vi "waitForRisEdgeTest.vi"(6 "stop":bool, 9 "delay(ticks)":u32) -> (3 "i":i32)   [LabVIEW 2014]
uses:
  <vilib>/eio/EIONode/EIONode.xnode
  <vilib>/rvi/eio/common/nirviEmuTemplateMethod_errors.vi
panel:
  in  "trigSelect":u16 format="%016b"
  in  "waitbeforeNextGo(Ticks)":u32 caption="waitBeforeNextGo(Ticks)"
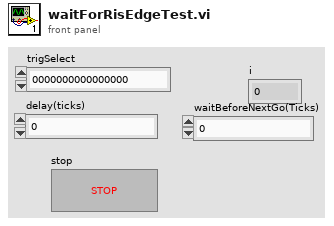
[diagram p1: front panel]
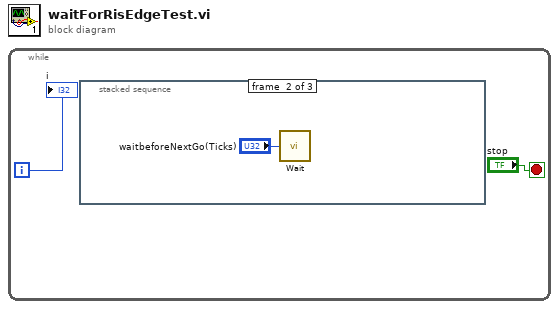
[diagram p0: block diagram]
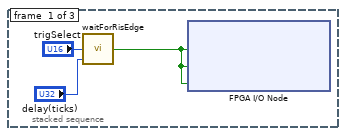
[diagram p2: hidden frame]
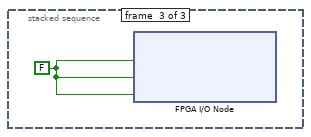
[diagram p3: hidden frame]
diagram:
  n1 = while {
    i -> [w1]
    stop <- "stop" stop-if-true
    n2 = stacked-sequence {
      frame #0 {
        n3 = call "waitForRisEdge.vi"("delay(ticks)"="delay(ticks)", "MCSSelectTrigger"="trigSelect") -> ("out"=w3:bool)  [unwired: 2 in, 1 out]
        n4 = xnode "FPGA I/O Node"("Connector1/DIO15"=w3, "Connector1/DIO9"=w3, "Connector1/DIO10"=w3) -> ()  [unwired: 3 in, 3 out]
      }
      frame #1 {
        n5 = call "Wait"("Count(Ticks)"="waitbeforeNextGo(Ticks)") -> ()  [unwired: 1 out]
      }
      frame #2 {
        w7 = FALSE ("Connector1/DIO15")
        n6 = xnode "FPGA I/O Node"("Connector1/DIO15"=w7, "Connector1/DIO9"=w7, "Connector1/DIO10"=w7) -> ()  [unwired: 3 in, 3 out]
      }
    }
    "i" <- w1
  }
